vi "Orca Flash Messanger.vi"(0 "Notifier Name":string, 2 "Camera Actions":T5, 5 "sCMOS Parameter":T3={"Value"=0.0, "Parameter"=4212128} {"Parameter" items=["SENSOR MODE"=4212128, "READOUT SPEED"=4211872, "READOUT DIRECTION"=4211904, "TRIGGER GLOBAL EXPOSURE"=2049680, "TRIGGER DELAY"=1066480, "SYNC READOUT SYSTEM BLANK"=1066528, "SENSOR COOLER"=2115248, "SENSOR COOLER STATUS"=2115280, "EXPOSURE TIME"=2049184, "DEFECT CORRECT MODE"=4670368, "BINNING"=4215968, "INTERNAL LINE SPEED"=4226000, "INTERNAL LINE INTERVAL"=4226016, "IMAGE PIXEL TYPE"=4343296, "NUMBER OF OUTPUT TRIGGER CONNECTOR"=1852320, "OUTPUT TRIGGER SOURCE[0]"=1852576, "OUTPUT TRIGGER SOURCE[1]"=1852832, "OUTPUT TRIGGER SOURCE[2]"=1853088, "OUTPUT TRIGGER POLARITY[0]"=1852592, "OUTPUT TRIGGER POLARITY[1]"=1852848, "OUTPUT TRIGGER POLARITY[2]"=1853104, "OUTPUT TRIGGER ACTIVE[0]"=1852608, "OUTPUT TRIGGER ACTIVE[1]"=1852864, "OUTPUT TRIGGER ACTIVE[2]"=1853120, "OUTPUT TRIGGER DELAY[0]"=1852624, "OUTPUT TRIGGER DELAY[1]"=1852880, "OUTPUT TRIGGER DELAY[2]"=1853136, "OUTPUT TRIGGER PERIOD[0]"=1852640, "OUTPUT TRIGGER PERIOD[1]"=1852896, "OUTPUT TRIGGER PERIOD[2]"=1853152, "OUTPUT TRIGGER KIND[0]"=1852656, "OUTPUT TRIGGER KIND[1]"=1852912, "OUTPUT TRIGGER KIND[2]"=1853168, "OUTPUT TRIGGER PRE HSYNC COUNT"=1852704, "OPM Trigger"=0]}, 7 "sCMOS ROI":T2, 9 "Path":path, 11 "# of frames":u32) -> (4 "Notifier Name Dup":string, 6 "Running?":bool, 8 "sCMOS Parameter":T3={"Value"=0.0, "Parameter"=4212128} {"Parameter" items=["SENSOR MODE"=4212128, "READOUT SPEED"=4211872, "READOUT DIRECTION"=4211904, "TRIGGER GLOBAL EXPOSURE"=2049680, "TRIGGER DELAY"=1066480, "SYNC READOUT SYSTEM BLANK"=1066528, "SENSOR COOLER"=2115248, "SENSOR COOLER STATUS"=2115280, "EXPOSURE TIME"=2049184, "DEFECT CORRECT MODE"=4670368, "BINNING"=4215968, "INTERNAL LINE SPEED"=4226000, "INTERNAL LINE INTERVAL"=4226016, "IMAGE PIXEL TYPE"=4343296, "NUMBER OF OUTPUT TRIGGER CONNECTOR"=1852320, "OUTPUT TRIGGER SOURCE[0]"=1852576, "OUTPUT TRIGGER SOURCE[1]"=1852832, "OUTPUT TRIGGER SOURCE[2]"=1853088, "OUTPUT TRIGGER POLARITY[0]"=1852592, "OUTPUT TRIGGER POLARITY[1]"=1852848, "OUTPUT TRIGGER POLARITY[2]"=1853104, "OUTPUT TRIGGER ACTIVE[0]"=1852608, "OUTPUT TRIGGER ACTIVE[1]"=1852864, "OUTPUT TRIGGER ACTIVE[2]"=1853120, "OUTPUT TRIGGER DELAY[0]"=1852624, "OUTPUT TRIGGER DELAY[1]"=1852880, "OUTPUT TRIGGER DELAY[2]"=1853136, "OUTPUT TRIGGER PERIOD[0]"=1852640, "OUTPUT TRIGGER PERIOD[1]"=1852896, "OUTPUT TRIGGER PERIOD[2]"=1853152, "OUTPUT TRIGGER KIND[0]"=1852656, "OUTPUT TRIGGER KIND[1]"=1852912, "OUTPUT TRIGGER KIND[2]"=1853168, "OUTPUT TRIGGER PRE HSYNC COUNT"=1852704, "OPM Trigger"=0]}, 10 "sCMOS ROI":T2, 15 "Image Ref":T1)   [LabVIEW 2025]
uses:
  Orca Flash Controls/Orca Flash Parameters.ctl
  Orca Flash Controls/Orca Flash Parameter List.ctl
  Orca Flash Controls/Orca Flash Actions.ctl
  Orca Flash Controls/Orca Flash ROI.ctl
  <vilib>/vision/Image Controls.llb/IMAQ Image.ctl
  Orca Flash Controls/Orca Flash Notifier Element.ctl
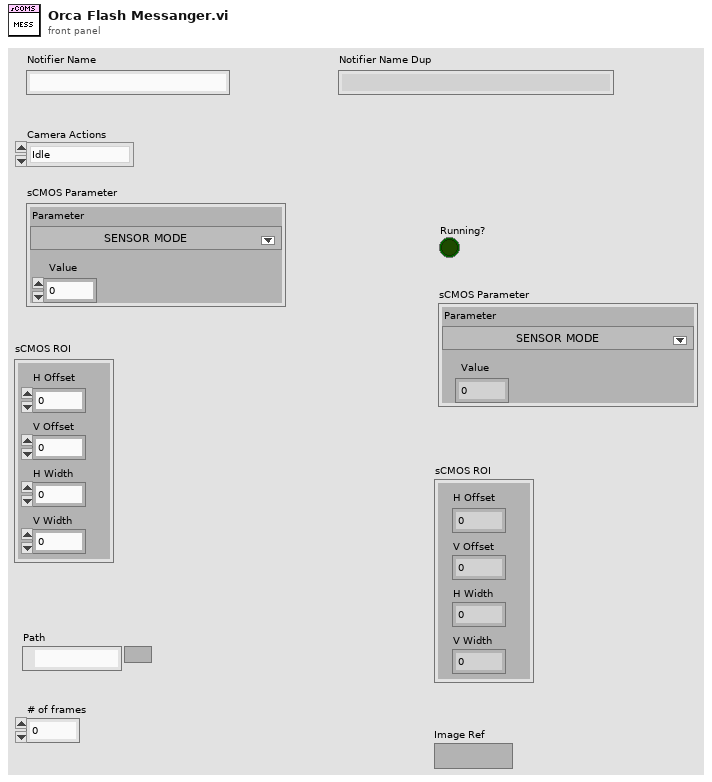
[diagram p1: front panel]
types:
  T1 = typedef "IMAQ Image.ctl" = refnum<image>
  T2 = typedef "Orca Flash ROI.ctl" = cluster{"H Offset":i32, "V Offset":i32, "H Width":i32, "V Width":i32}
  T3 = typedef "Orca Flash Parameters.ctl" = cluster{"Value":dbl, "Parameter":T4}
  T4 = typedef "Orca Flash Parameter List.ctl" = u32
  T5 = typedef "Orca Flash Actions.ctl" = enum16{"Idle", "Preview", "Record", "Record Settings", "Set Param", "Get Param", "Set ROI", "Get ROI", "Trigger Source", "Trigger Type", "Progessive Mode", "Area Mode", "Status", "Quit"}
  T6 = typedef "Orca Flash Notifier Element.ctl" = cluster{"Camera Actions":T5, "Received?":bool, "Running?":bool, "sCMOS Parameter":T3, "sCMOS ROI":T2, "Save Path":path, "# of frames":u32, "Image Ref":T1}
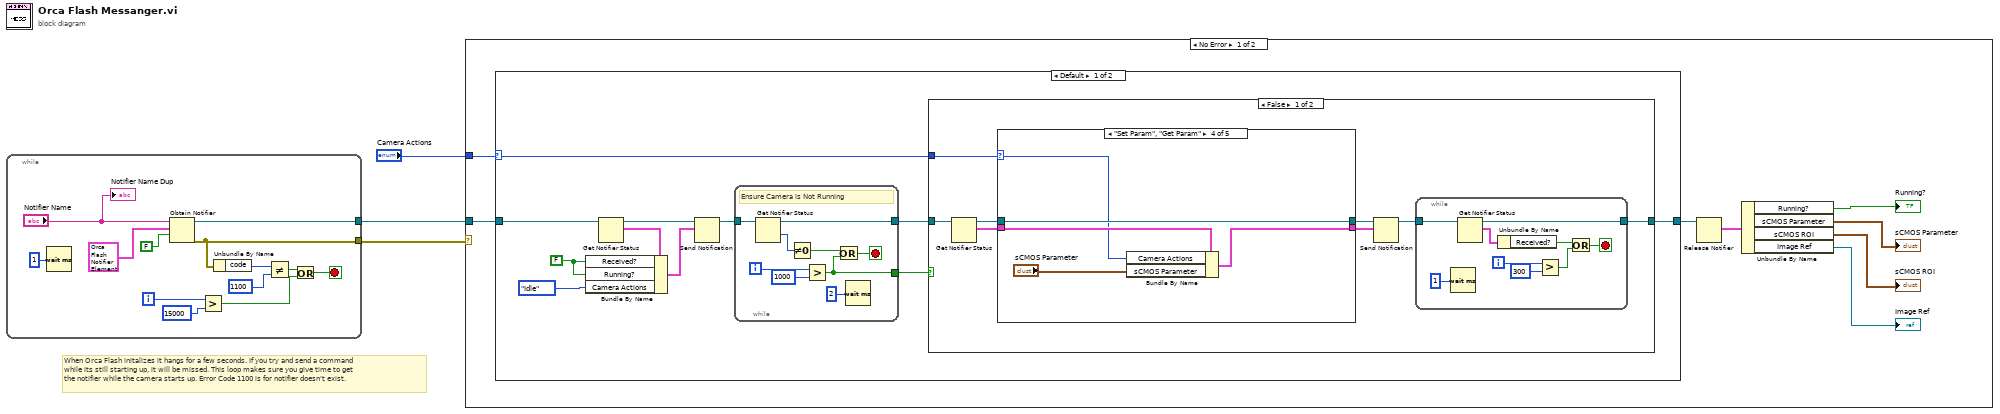
[diagram p0: block diagram]
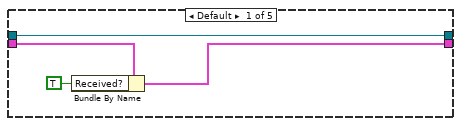
[diagram p2: hidden frame]
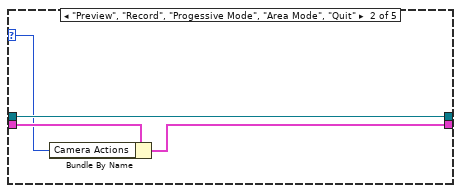
[diagram p3: hidden frame]
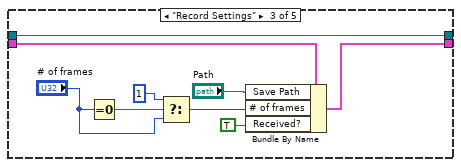
[diagram p4: hidden frame]
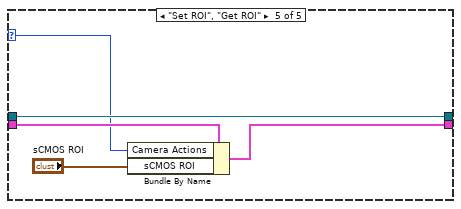
[diagram p5: hidden frame]
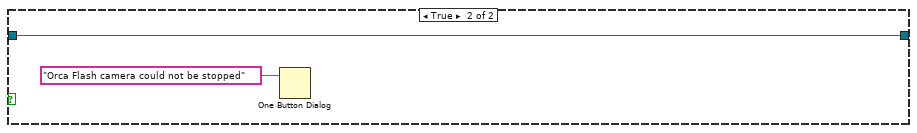
[diagram p6: hidden frame]
diagram:
  # "When Orca Flash initalizes it hangs for a few seconds. If you try and send a command\nwhile its still starting up, it will be missed. This loop makes sure you give time to get\nthe notifier while the camera starts up. Error Code 1100 is for notifier doesn't exist."
  n1 = while {
    tunnel: [w5] -> w2
    tunnel: [w4] -> w1
    i -> [w9]
    stop <- w6 stop-if-true
    n2 = Wait (ms)(milliseconds to wait=u32 1) -> ()  [unwired: 1 out]
    n3 = Obtain Notifier(name (unnamed)="Notifier Name", notification data type=T6 {"Camera Actions"=enum."Idle", "Received?"=FALSE, "Running?"=FALSE, "sCMOS Parameter"={"Value"=0.0, "Parameter"=0}, "sCMOS ROI"={"H Offset"=0, "V Offset"=0, "H Width"=0, "V Width"=0}, "Save Path"=path "", "# of frames"=0, "Image Ref"=refnum} ("Camera Cluster"), create if not found? (T)=FALSE) -> (notifier out=w4:refnum<notifier>, error out=w5:errorcluster)  [unwired: 1 in, 1 out]
    n4 = Greater?(x=w9, y=15000) -> (0:w7:bool)
    n5 = Unbundle By Name(w5) -> ("code"=w13:i32)
    n6 = Not Equal?(x=w13, y=1100) -> (x != y?=w11:bool)
    n7 = Or(x=w11, y=w7) -> (x .or. y?=w6:bool)
    "Notifier Name Dup" <- "Notifier Name"
  }
  n8 = case shown="No Error" w2 {
    tunnel: w1 -> [w24 _]
    tunnel: "Camera Actions" -> [w18 _]
    frame No Error {
      n9 = case shown="Default" w18 {
        selector: w18 -> [w26 _]
        tunnel: w24 -> [w34 w91]
        tunnel: [w27 w91] -> w17
        frame Default {
          w32 = FALSE ("Received?")
          n10 = Get Notifier Status(notifier=w34) -> (notifier out=w35:refnum<notifier>, current notification=w33:T6)  [unwired: 1 in, 3 out]
          n11 = Bundle By Name(cluster=w33, "Received?"=w32, "Running?"=w32, "Camera Actions"=Orca_Flash_Actions."Idle") -> (w31:T6)
          n12 = Send Notification(notification=w31, notifier=w35) -> (notifier out=w30:refnum<notifier>)  [unwired: 1 in, 1 out]
          n13 = while {
            tunnel: w30 -> [w90]
            tunnel: [w89] -> w29
            tunnel: [w84] -> w28
            i -> [w86]
            stop <- w88 stop-if-true
            # "Ensure Camera is Not Running"
            n14 = Get Notifier Status(notifier=w90) -> (notifier out=w89:refnum<notifier>, # waiting=w83:i32)  [unwired: 1 in, 3 out]
            n15 = Not Equal To 0?(x=w83) -> (x != 0?=w82:bool)
            n16 = Greater?(x=w86, y=1000) -> (0:w84:bool)
            n17 = Or(x=w82, y=w84) -> (x .or. y?=w88:bool)
            n18 = Wait (ms)(milliseconds to wait=u32 2) -> ()  [unwired: 1 out]
          }
          n19 = case shown="False" w28 {
            tunnel: w29 -> [w43 w81]
            tunnel: [w36 w81] -> w27
            tunnel: w26 -> [w40 _]
            frame False {
              n20 = Get Notifier Status(notifier=w43) -> (notifier out=w42:refnum<notifier>, current notification=w41:T6)  [unwired: 1 in, 3 out]
              n21 = case shown="\"Set Param\", \"Get Param\"" w40 {
                selector: w40 -> [_ w57 _ w70 w75]
                tunnel: [w56 w59 w62 w72 w76] -> w39
                tunnel: w42 -> [w56 w59 w62 w72 w76]
                tunnel: w41 -> [w54 w60 w69 w74 w79]
                tunnel: [w53 w58 w63 w71 w77] -> w38
                frame Default {
                  n22 = Bundle By Name(cluster=w54, "Received?"=TRUE) -> (w53:T6)
                }
                frame "Preview", "Record", "Progessive Mode", "Area Mode", "Quit" {
                  n23 = Bundle By Name(cluster=w60, "Camera Actions"=w57) -> (w58:T6)
                }
                frame "Record Settings" {
                  n24 = Equal To 0?(x="# of frames") -> (x = 0?=w66:bool)
                  n25 = Select(t=u32 1, s=w66, f="# of frames") -> (s? t:f=w64:u32)
                  n26 = Bundle By Name(cluster=w69, "Save Path"="Path", "# of frames"=w64, "Received?"=TRUE) -> (w63:T6)
                }
                frame "Set Param", "Get Param" {
                  n27 = Bundle By Name(cluster=w74, "Camera Actions"=w70, "sCMOS Parameter"="sCMOS Parameter") -> (w71:T6)
                }
                frame "Set ROI", "Get ROI" {
                  n28 = Bundle By Name(cluster=w79, "Camera Actions"=w75, "sCMOS ROI"="sCMOS ROI") -> (w77:T6)
                }
              }
              n29 = Send Notification(notification=w38, notifier=w39) -> (notifier out=w37:refnum<notifier>)  [unwired: 1 in, 1 out]
              n30 = while {
                tunnel: w37 -> [w52]
                tunnel: [w44] -> w36
                i -> [w49]
                stop <- w45 stop-if-true
                n31 = Wait (ms)(milliseconds to wait=u32 1) -> ()  [unwired: 1 out]
                n32 = Get Notifier Status(notifier=w52) -> (notifier out=w44:refnum<notifier>, current notification=w51:T6)  [unwired: 1 in, 3 out]
                n33 = Unbundle By Name(w51) -> ("Received?"=w50:bool)
                n34 = Greater?(x=w49, y=300) -> (0:w47:bool)
                n35 = Or(x=w50, y=w47) -> (x .or. y?=w45:bool)
              }
            }
            frame True {
              n36 = One Button Dialog(message="Orca Flash camera could not be stopped") -> ()  [unwired: 1 in, 1 out]
            }
          }
        }
        frame "Status" {
        }
      }
      n37 = Release Notifier(notifier=w17) -> (last notification=w23:T6)  [unwired: 2 in, 2 out]
      n38 = Unbundle By Name(w23) -> ("Running?"=→"Running?":bool, "sCMOS Parameter"=→"sCMOS Parameter":T3, "sCMOS ROI"=→"sCMOS ROI":T2, "Image Ref"=→"Image Ref":T1)
    }
    frame Error {
    }
  }
